vi "Extract Tar Archive.vi"(8 "error in (no error)":errorcluster, 11 "File":path=path "") -> (0 "error out":errorcluster)   [LabVIEW 2020, in "binary_installation_tools.lvlib"]
uses:
  binary_installation_tools.lvlib
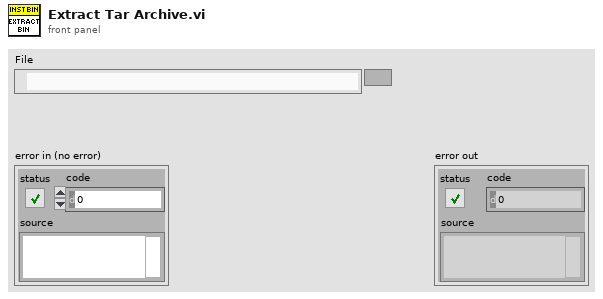
[diagram p1: front panel]
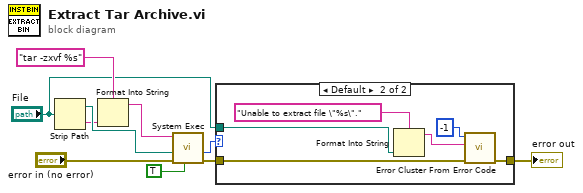
[diagram p0: block diagram]
diagram:
  n1 = Strip Path(path="File") -> (stripped path=w10:path, name=w8:string)
  n2 = Format Into String(format string="tar -zxvf %s", w8) -> (resulting string=w7:string)  [unwired: 2 in, 1 out]
  n3 = call <vilib>:"System Exec.vi"("run minimized? (F)"=TRUE, "error in (no error)"="error in (no error)", "working directory"=w10, "command line"=w7) -> ("error out"=w3:errorcluster, "return code"=w5:i32)  [unwired: 4 in, 2 out]
  n4 = case shown="Default" w5 {
    tunnel: [w11 w16] -> w4
    tunnel: w3 -> [w11 w17]
    tunnel: "File" -> [_ w15]
    frame 0 {
    }
    frame Default {
      n5 = Format Into String(format string="Unable to extract file \"%s\".", w15) -> (resulting string=w13:string)  [unwired: 2 in, 1 out]
      n6 = call <vilib>:"Error Cluster From Error Code.vi"("error in (no error)"=w17, "error message (\"\")"=w13, "error code (0)"=-1) -> ("error out"=w16:errorcluster)  [unwired: 6 in]
    }
  }
  "error out" <- w4
